vi "AB - Abort Motion.vi"(8 "error in":errorcluster, 11 "Address / Port":i16=1 min=1 max=31 step=1) -> (0 "error out":errorcluster)   [LabVIEW 2014]
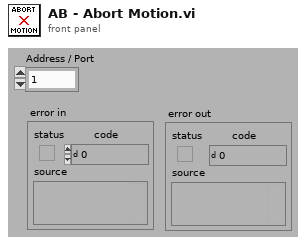
[diagram p1: front panel]
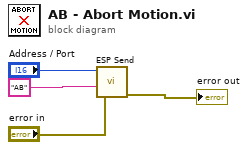
[diagram p0: block diagram]
diagram:
  n1 = call "ESP Send.vi"("error in"="error in", "Command String"="AB" ("Substring"), "Address / Port"="Address / Port") -> ("error out"=→"error out":errorcluster)  [unwired: 3 in, 1 out]
